vi "shuffle_dbl.vi"(1 "Array IN":dbl[][](array[numeric])) -> (0 "Array OUT":dbl[][](array[numeric]))   [LabVIEW 2015, in "oskar_tools.lvlib"]
uses:
  oskar_tools.lvlib
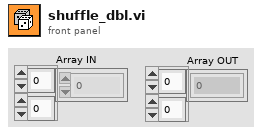
[diagram p1: front panel]
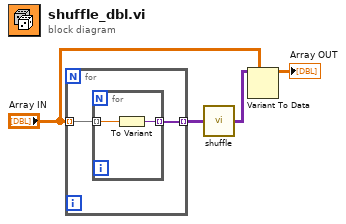
[diagram p0: block diagram]
diagram:
  n1 = for {
    tunnel: "Array IN" -> [w6] mode=indexing
    tunnel: [w5] -> w4 mode=indexing
    n2 = for {
      tunnel: w6 -> [w8] mode=indexing
      tunnel: [w7] -> w5 mode=indexing
      n3 = To Variant(anything=w8) -> (Variant=w7:variant)
    }
  }
  n4 = call "shuffle.vi"("Array IN"=w4) -> ("Array OUT"=w3:variant[][])
  n5 = Variant To Data(type="Array IN", Variant=w3) -> (data=→"Array OUT":dbl[][])  [unwired: 1 in, 1 out]
